vi "WS1021 Multi DUT VPI DeltaC.vi"(8 "Error In":errorcluster, 11 "VPI Input":string[][](table)) -> (0 "Error Out":errorcluster, 1 "VPI % Delta C":string[](array[string]), 2 "VPI Total Delta C (fF)":string[](array[string]), 3 "VPI Delta C R2 (fF)":string[](array[string]), 5 "VPI Delta C R3 (fF)":string[](array[string]))   [LabVIEW 2017]
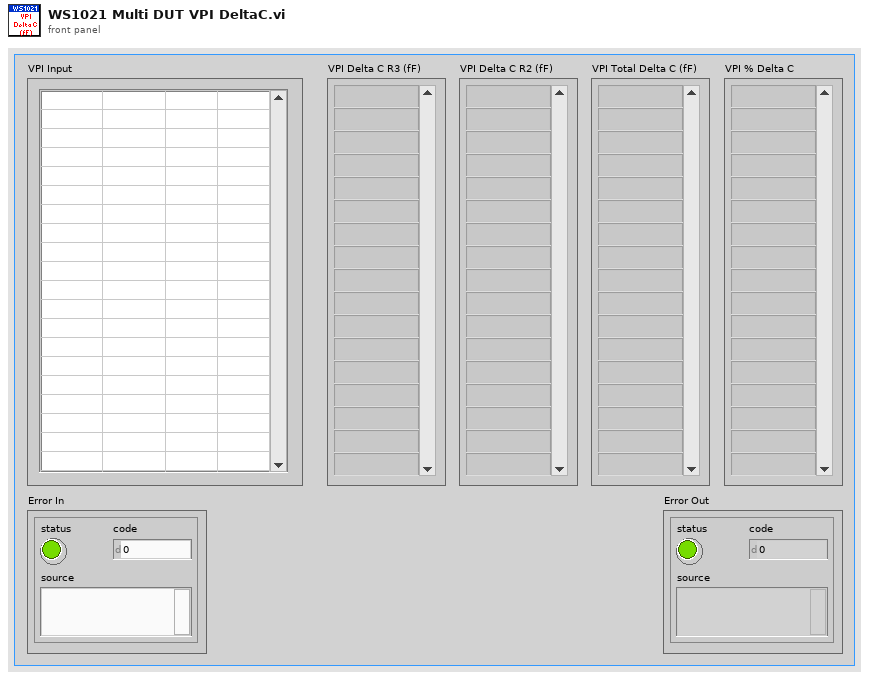
[diagram p1: front panel]
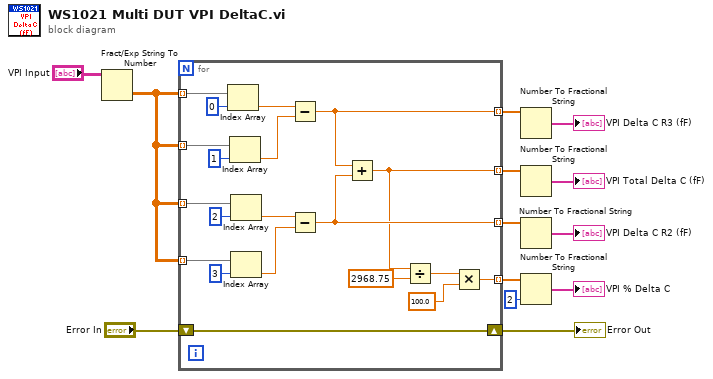
[diagram p0: block diagram]
diagram:
  n1 = Fract/Exp String To Number(string="VPI Input") -> (number=w12:dbl[][])  [unwired: 3 in, 1 out]
  n2 = for {
    tunnel: w12 -> [w33] mode=indexing
    tunnel: w12 -> [w30] mode=indexing
    tunnel: w12 -> [w23] mode=indexing
    tunnel: w12 -> [w22] mode=indexing
    tunnel: [w21] -> w11 mode=indexing
    tunnel: [w20] -> w7 mode=indexing
    tunnel: [w19] -> w9 mode=indexing
    tunnel: [w15] -> w5 mode=indexing
    shift-right: [w14] -> w2
    shift-left: "Error In" -> [w14]
    n3 = Index Array(array=w33, index=0) -> (element=w29:dbl)
    n4 = Index Array(array=w30, index=1) -> (element=w28:dbl)
    n5 = Index Array(array=w23, index=2) -> (element=w25:dbl)
    n6 = Index Array(array=w22, index=3) -> (element=w24:dbl)
    n7 = Subtract(x=w29, y=w28) -> (x-y=w21:dbl)
    n8 = Subtract(x=w25, y=w24) -> (x-y=w20:dbl)
    n9 = Add(x=w21, y=w20) -> (x+y=w19:dbl)
    n10 = Divide(x=w19, y=2968.75) -> (x/y=w18:dbl)
    n11 = Multiply(x=w18, y=100.0) -> (x*y=w15:dbl)
  }
  "Error Out" <- w2
  n12 = Number To Fractional String(number=w11) -> (F-format string=→"VPI Delta C R3 (fF)":string[])  [unwired: 3 in]
  n13 = Number To Fractional String(number=w9) -> (F-format string=→"VPI Total Delta C (fF)":string[])  [unwired: 3 in]
  n14 = Number To Fractional String(number=w7) -> (F-format string=→"VPI Delta C R2 (fF)":string[])  [unwired: 3 in]
  n15 = Number To Fractional String(number=w5, precision (6)=i16 2) -> (F-format string=→"VPI % Delta C":string[])  [unwired: 2 in]
